vi "Koch.vi"(9 "x_coord":dbl[](array[numeric]), 10 "y_coord":dbl[](array[numeric]), 11 "depth":dbl) -> (2 "y_coord 2":dbl[](array[numeric]), 3 "x_coord 2":dbl[](array[numeric]))   [LabVIEW 2024]
panel:
  out "depth 2":dbl
  out "XY Graph":cluster{"X":dbl, "Y":dbl}[](graph)
  in  "length":dbl
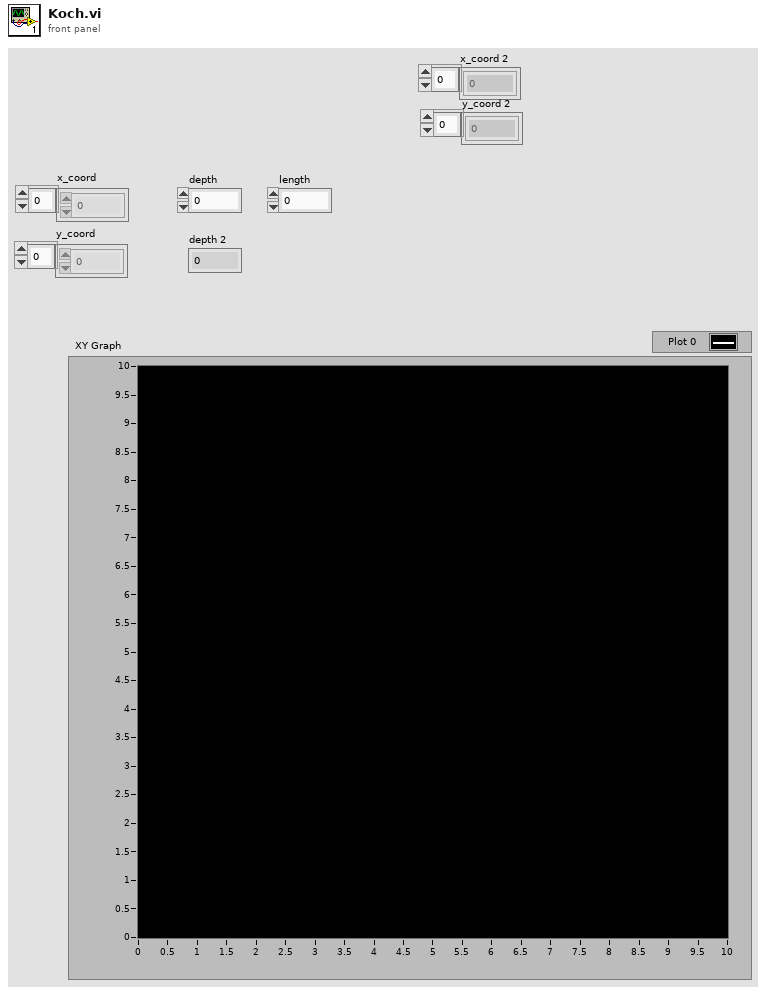
[diagram p1: front panel]
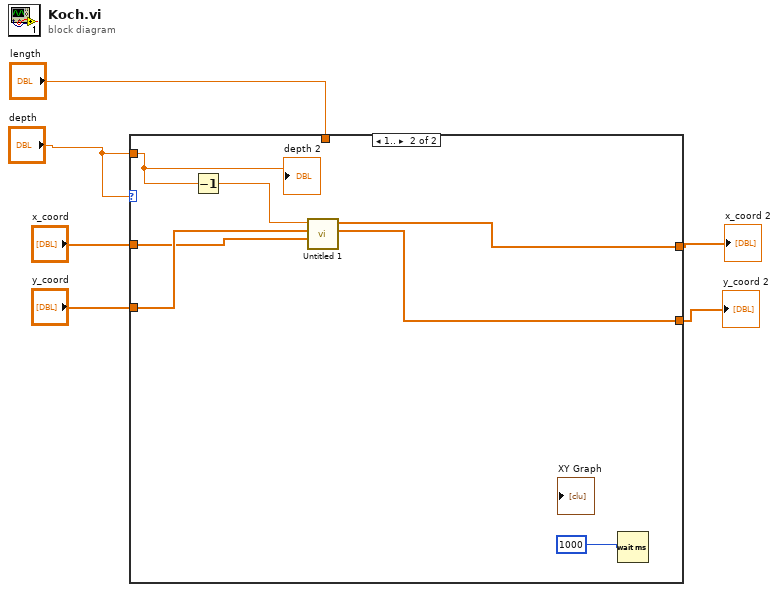
[diagram p0: block diagram]
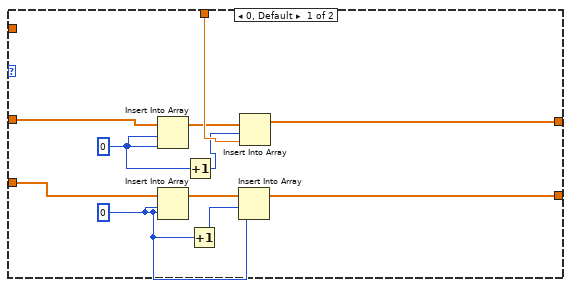
[diagram p2: hidden frame]
diagram:
  n1 = case shown="1.." "depth" {
    tunnel: "x_coord" -> [w17 w23]
    tunnel: "y_coord" -> [w16 w24]
    tunnel: "length" -> [w15 _]
    tunnel: [w8 w22] -> w3
    tunnel: [w7 w21] -> w2
    tunnel: "depth" -> [_ w20]
    frame 0, Default {
      w9 = 0
      w14 = 0
      n2 = Insert Into Array(array=w17, index=w14, new element=w14) -> (w12:dbl[])
      n3 = Insert Into Array(array=w16, index=w9, new element=w9) -> (w11:dbl[])
      n4 = Increment(x=w14) -> (x+1=w13:i32)
      n5 = Increment(x=w9) -> (x+1=w10:i32)
      n6 = Insert Into Array(array=w11, index=w10, new element=w9) -> (w7:dbl[])
      n7 = Insert Into Array(array=w12, index=w13, new element=w15) -> (w8:dbl[])
    }
    frame 1.. {
      n8 = Decrement(x=w20) -> (x-1=w18:dbl)
      n9 = call "Untitled 1.vi"("x_coord"=w23, "y_coord"=w24, "depth"=w18) -> ("y_coord 2"=w21:dbl[], "x_coord 2"=w22:dbl[])  [unwired: 7 in]
      n10 = Wait (ms)(milliseconds to wait=u32 1000) -> ()  [unwired: 1 out]
      "depth 2" <- w20
    }
  }
  "x_coord 2" <- w3
  "y_coord 2" <- w2
